vi "enteringTargetState.vi"(8 "error in (no error)":errorcluster, 11 "statemachine in":refnum<class "statemachine.lvclass">) -> (0 "error out":errorcluster, 3 "statemachine out":refnum<class "statemachine.lvclass">)   [LabVIEW 2020, in "eos.lvlib" / "statemachine.lvclass"]
uses:
  statemachine.lvclass
  statemachine.lvclass/statemachine.ctl
  interfaces/state/state.lvclass
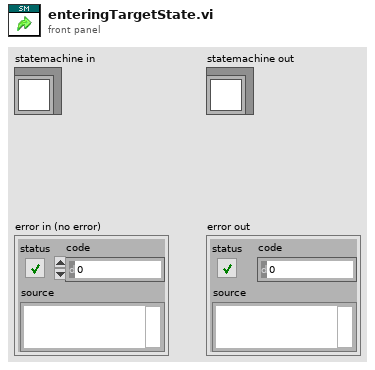
[diagram p1: front panel]
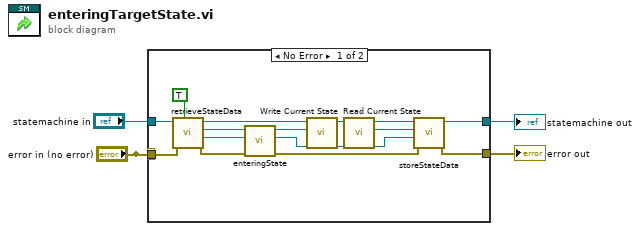
[diagram p0: block diagram]
diagram:
  n1 = case shown="No Error" "error in (no error)" {
    selector: "error in (no error)" -> [_ w21]
    tunnel: [w16 w21] -> w3
    tunnel: [w12 w20] -> w2
    tunnel: "statemachine in" -> [w19 w20]
    tunnel: "error in (no error)" -> [w15 _]
    frame No Error {
      n2 = call "retrieveStateData.vi"("Target? (F)"=TRUE, "error in (no error)"=w15, "statemachine in"=w19) -> ("error out"=w17:errorcluster, "State Data"=w14:refnum<class "data.lvclass">, "State"=w9:refnum<class "state.lvclass">, "statemachine out"=w10:refnum<class "statemachine.lvclass">)  [unwired: 5 in]
      n3 = call-dynamic "enteringState.vi"("error in (no error)"=w17, "State Data in"=w14, "Target state in"=w9) -> ("error out"=w18:errorcluster, "State Data out"=w11:refnum<class "data.lvclass">, "Target state out"=w8:refnum<class "state.lvclass">)  [unwired: 6 in]
      n4 = call "Write Current State.vi"("Current State"=w8, "statemachine in"=w10) -> ("statemachine out"=w6:refnum<class "statemachine.lvclass">)  [unwired: 9 in]
      n5 = call "Read Current State.vi"("statemachine in"=w6) -> ("Current State"=w7:refnum<class "state.lvclass">, "statemachine out"=w5:refnum<class "statemachine.lvclass">)  [unwired: 9 in]
      n6 = call "storeStateData.vi"("error in (no error)"=w18, "State Data"=w11, "Current State"=w7, "statemachine in"=w5) -> ("error out"=w16:errorcluster, "statemachine out"=w12:refnum<class "statemachine.lvclass">)  [unwired: 5 in, 1 out]
    }
    frame Error {
    }
  }
  "statemachine out" <- w2
  "error out" <- w3
